vi "Test_Combo Filter.vi"(8 "error in":errorcluster, 9 "aggregation method":T1, 10 "match behavior":T2, 11 "directory":path=path "C:/Users/Colin/Documents/software_projects/labview/glog/logs/test") -> (0 "error out":errorcluster, 3 "failure info":T3 {"Log Record"."timestamp" format="%<%x %.3X>T"})   [LabVIEW 2018]
uses:
  src/api/logger_class/Failure Information.ctl
  src/api/logger_class/Log Record.ctl
  src/api/logger_class/Internal Log Levels.ctl
  src/api/extension/filter_interface/Match Behavior.ctl
  src/api/extension/filter_interface/Aggregation Method.ctl
  src/api/logger_class/Log Levels.ctl
  src/api/configuration/filters/regex_filter/Regex.lvclass
  C:/Users/Colin/Documents/software_projects/labview/glog/src/api/extension/filter_interface/Filter.lvclass
  src/api/configuration/filters/combination_filter/Combination.lvclass
  src/api/configuration/handlers/file_handler/File Handler.lvclass
  C:/Users/Colin/Documents/software_projects/labview/glog/src/api/extension/formatting_handler_interface/Formatting Handler.lvclass
  src/api/configuration/filters/regex_filter/New (Element).vi
  src/api/logger_class/Log (Parts).vi
  src/api/logger_class/Logger.lvclass
  src/api/GLog.lvlib
panel:
  # "Connector Pane"
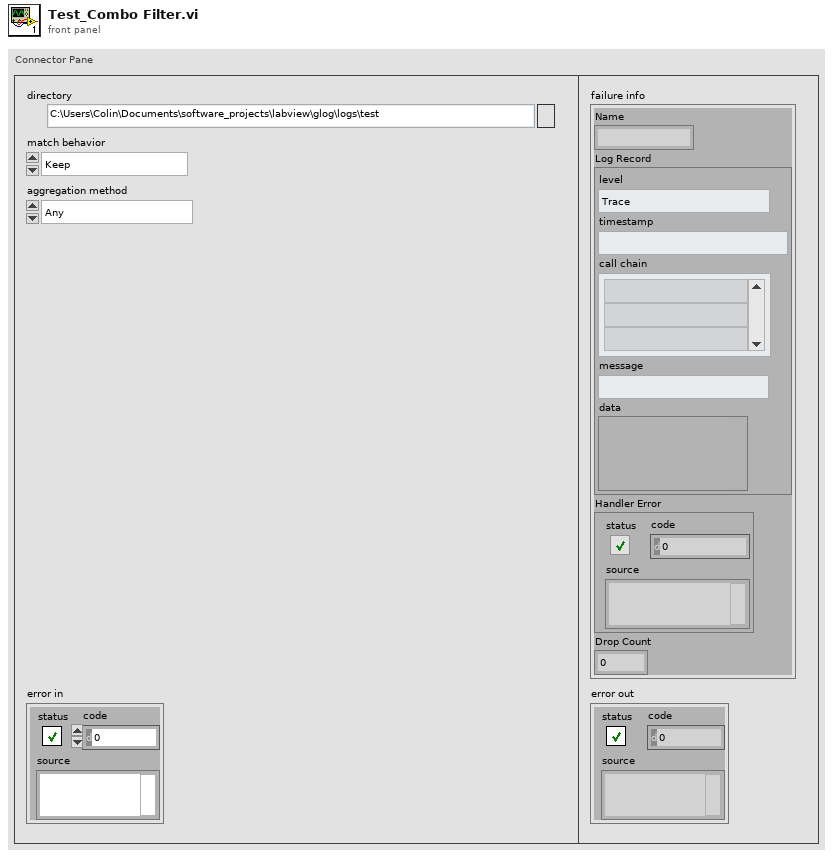
[diagram p1: front panel]
types:
  T1 = typedef "GLog.lvlib/Aggregation Method.ctl" = enum16{"Any", "Only", "All", "None"}
  T2 = typedef "GLog.lvlib/Match Behavior.ctl" = enum16{"Keep", "Discard"}
  T3 = typedef "GLog.lvlib/Logger.lvclass/Failure Information.ctl" = cluster{"Name":string, "Log Record":T4, "Handler Error":errorcluster, "Drop Count":u32}
  T4 = typedef "GLog.lvlib/Logger.lvclass/Log Record.ctl" = cluster{"level":T5, "timestamp":timestamp, "call chain":string[], "message":string, "data":variant}
  T5 = typedef "GLog.lvlib/Logger.lvclass/Internal Log Levels.ctl" = enum16{"Trace", "Debug", "Info", "Warning", "Error", "Critical", "Internal"}
  T6 = typedef "GLog.lvlib/Logger.lvclass/Log Levels.ctl" = enum16{"Trace", "Debug", "Info", "Warning", "Error", "Critical"}
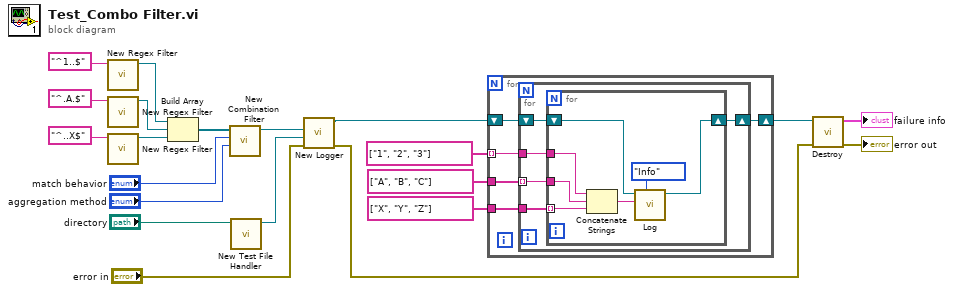
[diagram p0: block diagram]
diagram:
  n1 = call-poly "New Regex Filter.vi"("regex string"="^1..$") -> ("regex out"=w18:refnum<class "Regex.lvclass">)  [unwired: 9 in, 1 out]
  n2 = call-poly "New Regex Filter.vi"("regex string"="^.A.$") -> ("regex out"=w17:refnum<class "Regex.lvclass">)  [unwired: 9 in, 1 out]
  n3 = call-poly "New Regex Filter.vi"("regex string"="^..X$") -> ("regex out"=w16:refnum<class "Regex.lvclass">)  [unwired: 9 in, 1 out]
  n4 = Build Array(w18, w17, w16) -> (w12:refnum<class "Regex.lvclass">[])
  n5 = call "New Combination Filter.vi"("aggregation method (any)"="aggregation method", "match behavior (keep)"="match behavior", "sub-filters"=w12) -> ("aggregate filter"=w1:refnum<class "Combination.lvclass">)  [unwired: 8 in]
  n6 = call "New Test File Handler.vi"("log directory"="directory") -> ("test file handler"=w11:refnum<class "File Handler.lvclass">)  [unwired: 10 in]
  n7 = call "New Logger.vi"("error in (no error)"="error in", "log handler (file handler)"=w11, "log filter (none)"=w1) -> ("error out"=w5:errorcluster, "logger"=w7:refnum<class "Logger.lvclass">)  [unwired: 7 in]
  n8 = for {
    tunnel: string[] ["1", "2", "3"] -> [w26] mode=indexing
    tunnel: string[] ["A", "B", "C"] -> [w25]
    tunnel: string[] ["X", "Y", "Z"] -> [w24]
    shift-right: [w22] -> w6
    shift-left: w7 -> [w23]
    n9 = for {
      tunnel: w26 -> [w31]
      tunnel: w25 -> [w30] mode=indexing
      tunnel: w24 -> [w29]
      shift-right: [w27] -> w22
      shift-left: w23 -> [w28]
      n10 = for {
        tunnel: w31 -> [w38]
        tunnel: w30 -> [w37]
        tunnel: w29 -> [w36] mode=indexing
        shift-right: [w32] -> w27
        shift-left: w28 -> [w33]
        n11 = Concatenate Strings(w38, w37, w36) -> (w35:string)
        n12 = call-poly "Log.vi"("log level"=Log_Levels."Info", "message"=w35, "logger in"=w33) -> ("logger out"=w32:refnum<class "Logger.lvclass">)  [unwired: 8 in]
      }
    }
  }
  n13 = call "Destroy.vi"("error in (no error)"=w5, "logger in"=w6) -> ("error out"=→"error out":errorcluster, "failure info"=→"failure info":T3)  [unwired: 8 in]
